vi "Get GE 5565PIORC.vi"(11 "GE Reflective Memory in":refnum<class "GE Reflective Memory Transceiver.lvclass">) -> (2 "GE 5565PIORC":refnum<class "GE 5565PIORC.lvclass">, 3 "GE Reflective Memory out":refnum<class "GE Reflective Memory Transceiver.lvclass">)   [LabVIEW 2017, in "GE Reflective Memory Transceiver.lvlib" / "GE Reflective Memory Transceiver.lvclass"]
uses:
  GE Reflective Memory Transceiver.lvclass
  <vilib>/NI/GE Reflective Memory Driver/GE 5565PIORC.lvclass
  GE Reflective Memory Transceiver.lvclass/GE Reflective Memory Transceiver.ctl
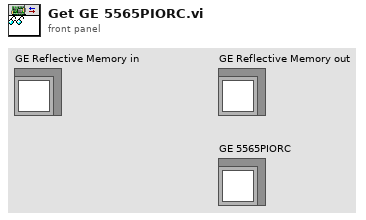
[diagram p1: front panel]
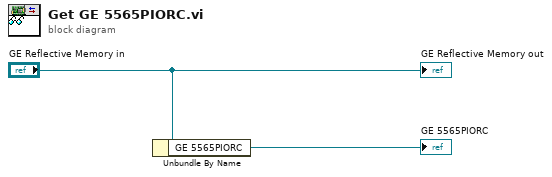
[diagram p0: block diagram]
diagram:
  n1 = Unbundle By Name("GE Reflective Memory in") -> ("GE 5565PIORC"=→"GE 5565PIORC":refnum<class "GE 5565PIORC.lvclass">)
  "GE Reflective Memory out" <- "GE Reflective Memory in"
